vi "Add Channels to Task.vi"(7 "TimingEngine":T1, 8 "error in":errorcluster, 9 "Chassis Name":string, 10 "Timing Grp":refnum<class "TimingGrp.lvclass">, 11 "DAQ Task":refnum<class "DAQ Task.lvclass">) -> (0 "error out":errorcluster, 3 "DAQ Task":refnum<class "DAQ Task.lvclass">)   [LabVIEW 2018, in "Data Acquisition.lvlib" / "DAQ Task.lvclass"]
uses:
  DAQ Task.lvclass
  Cfg Grandmaster/Class Timing Group/TimingGrp.lvclass
  Common/Controls/TE_Designator.ctl
  Measurements/Class Channel/Channel.lvclass
  DAQ Task.lvclass/DAQ Task.ctl
  Cfg Grandmaster/Class Timing Group/Read ChanGroups.vi
  Cfg Grandmaster/Class Chan Group/Read GroupChans.vi
  Measurements/Class Channel/Read Device.vi
  Cfg Grandmaster/Class Chan Group/ChanGrp.lvclass
  <resource>/objmgr/daqmx.rc
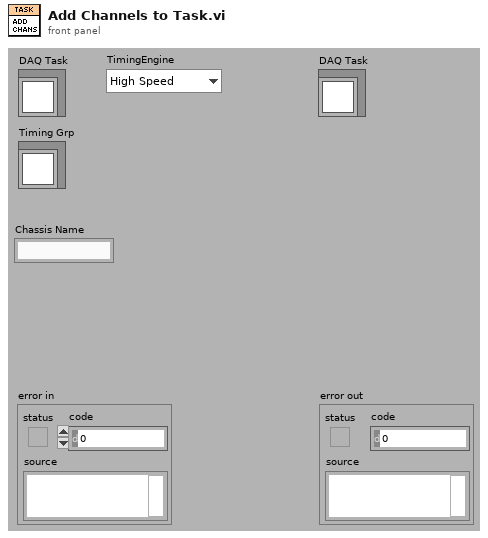
[diagram p1: front panel]
types:
  T1 = typedef "TE_Designator.ctl" = enum16{"High Speed", "Low Speed"}
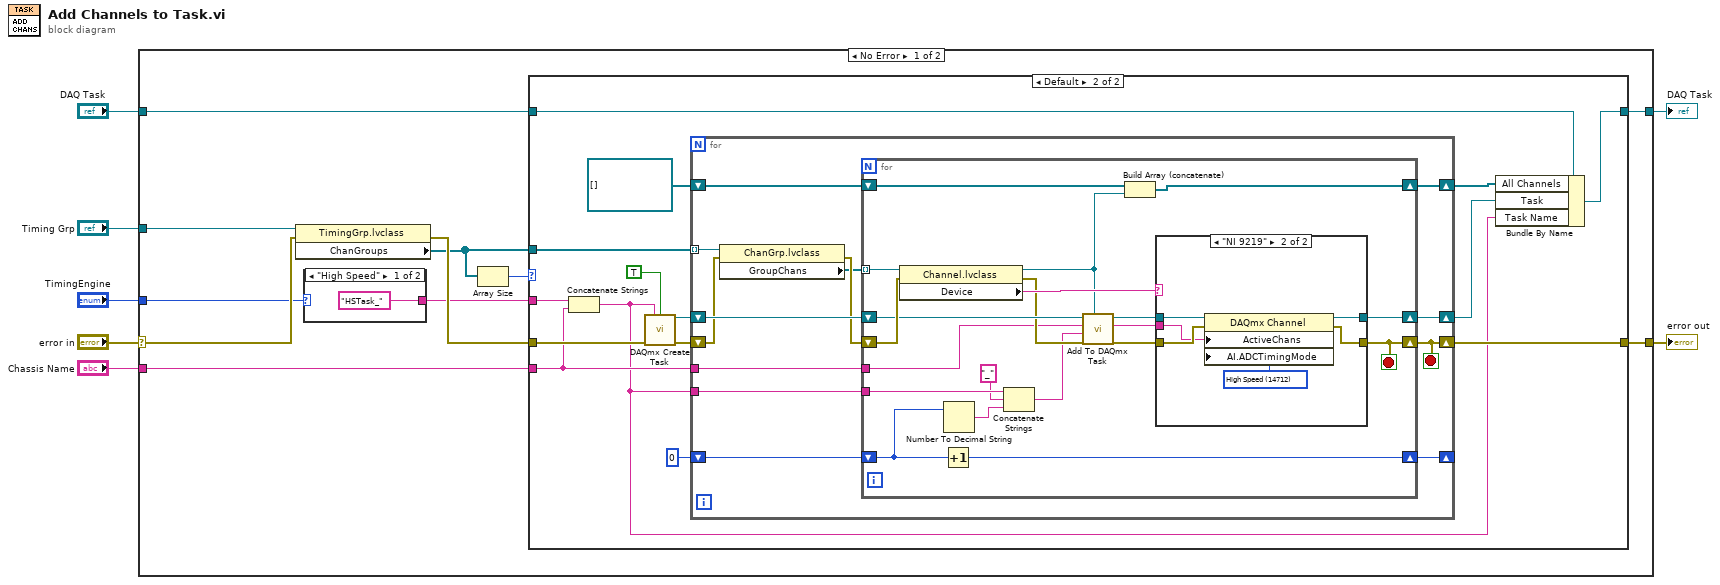
[diagram p0: block diagram]
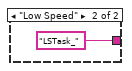
[diagram p4: hidden frame]
diagram:
  n1 = case shown="No Error" "error in" {
    selector: "error in" -> [w12 w80]
    tunnel: [w18 w79] -> w7
    tunnel: "Timing Grp" -> [w17 _]
    tunnel: "DAQ Task" -> [w14 w79]
    tunnel: [w13 w80] -> w4
    tunnel: "TimingEngine" -> [w9 _]
    tunnel: "Chassis Name" -> [w8 _]
    frame No Error {
      n2 = property class="TimingGrp.lvclass"(reference=w17, error in=w12) -> (error out=w16:errorcluster, "ChanGroups"=w11:refnum<class "ChanGrp.lvclass">[])  [unwired: 1 out]
      n3 = case shown="\"High Speed\"" w9 {
        tunnel: ["HSTask_" "LSTask_"] -> w15
        frame "High Speed" {
        }
        frame "Low Speed" {
        }
      }
      n4 = Array Size(array=w11) -> (size(s)=w10:i32)
      n5 = case shown="Default" w10 {
        tunnel: [w20 w35] -> w18
        tunnel: w16 -> [w19 w28]
        tunnel: w15 -> [_ w27]
        tunnel: w14 -> [w20 w26]
        tunnel: w8 -> [_ w25]
        tunnel: [w19 w24] -> w13
        tunnel: w11 -> [_ w23]
        frame 0 {
        }
        frame Default {
          n6 = Concatenate Strings(w27, w25) -> (w21:string)
          n7 = call <vilib>:"DAQmx Create Task.vi"("new task name"=w21, "auto cleanup"=TRUE, "error in"=w28) -> ("task out"=w33:refnum<k21>, "error out"=w34:errorcluster)  [unwired: 11 in]
          n8 = for {
            shift-right: [w41] -> w24
            shift-left: w34 -> [w38]
            shift-right: [w47] -> w22
            shift-left: w33 -> [w48]
            tunnel: w21 -> [w46]
            tunnel: w25 -> [w45]
            shift-right: [w43] -> _
            shift-left: 0 -> [w44]
            shift-right: [w40] -> w29
            shift-left: refnum<class "Channel.lvclass">[] [] -> [w42]
            tunnel: w23 -> [w39] mode=indexing
            stop <- w41 stop-if-true
            n9 = property class="ChanGrp.lvclass"(reference=w39, error in=w38) -> (error out=w37:errorcluster, "GroupChans"=w36:refnum<class "Channel.lvclass">[])  [unwired: 1 out]
            n10 = for {
              tunnel: w36 -> [w62] mode=indexing
              shift-right: [w67] -> w47
              shift-left: w48 -> [w59]
              shift-right: [w49] -> w41
              shift-left: w37 -> [w61]
              tunnel: w46 -> [w66]
              tunnel: w45 -> [w55]
              shift-right: [w68] -> w43
              shift-left: w44 -> [w65]
              shift-right: [w50] -> w40
              shift-left: w42 -> [w52]
              stop <- w49 stop-if-true
              n11 = property class="Channel.lvclass"(reference=w62, error in=w61) -> (reference out=w51:refnum<class "Channel.lvclass">, error out=w58:errorcluster, "Device"=w60:string)
              n12 = Increment(x=w65) -> (x+1=w68:i32)
              n13 = Number To Decimal String(number=w65) -> (decimal integer string=w64:string)  [unwired: 1 in]
              n14 = Concatenate Strings(w66, "_" ("string"), w64) -> (w54:string)
              n15 = call-dynamic "Add To DAQmx Task.vi"("Channel in"=w51, "error in (no error)"=w58, "Scale Name"=w54, "Chassis Name"=w55, "task in"=w59) -> ("error out"=w56:errorcluster, "Phys Chan Added"=w53:string, "task out"=w57:refnum<k21>)  [unwired: 4 in]
              n16 = Build Array (concatenate)(w52, w51) -> (w50:refnum<class "Channel.lvclass">[])
              n17 = case shown="\"NI 9219\"" w60 {
                tunnel: w57 -> [w69 w76]
                tunnel: w56 -> [w70 w75]
                tunnel: [w69 w74] -> w67
                tunnel: [w70 w73] -> w49
                tunnel: w53 -> [_ w72]
                frame "False", Default {
                }
                frame "NI 9219" {
                  w71 = 14712 items=["High Resolution"=10195, "High Speed"=14712, "Best 50 Hz Rejection"=14713, "Best 60 Hz Rejection"=14714, "Custom"=10137] ("AI.ADCTimingMode")
                  n18 = property class="DAQmx Channel"(reference=w76, error in=w75, "ActiveChans"=w72, "AI.ADCTimingMode"=w71) -> (reference out=w74:refnum<k21>, error out=w73:errorcluster)
                }
              }
            }
          }
          n19 = Bundle By Name(cluster=w26, "All Channels"=w29, "Task"=w22, "Task Name"=w21) -> (w35:refnum<class "DAQ Task.lvclass">)
        }
      }
    }
    frame Error {
    }
  }
  "error out" <- w4
  "DAQ Task" <- w7
